vi "LED_Scaled_Output.vi"(8 "Number of LEDs":i32=8, 9 "Range Bottom":dbl, 10 "Range Top":dbl=10.0, 11 "Sensor Input":dbl) -> (1 "Out of Range":bool, 3 "Output (bool)":bool[](array[boolean]), 4 "LEDs to light":dbl, 6 "Resolution":dbl)   [LabVIEW 2013]
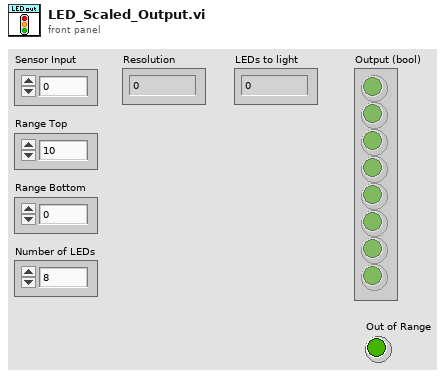
[diagram p1: front panel]
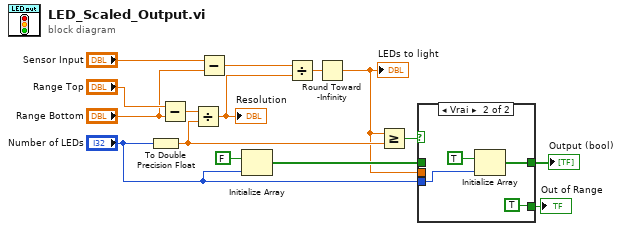
[diagram p0: block diagram]
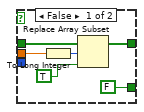
[diagram p2: hidden frame]
diagram:
  n1 = To Double Precision Float(number="Number of LEDs") -> (double precision float=w8:dbl)
  n2 = Subtract(x="Range Top", y="Range Bottom") -> (x-y=w13:dbl)
  n3 = Divide(x=w13, y=w8) -> (x/y=w12:dbl)
  "Resolution" <- w12
  n4 = Subtract(x="Sensor Input", y="Range Bottom") -> (x-y=w2:dbl)
  n5 = Initialize Array(FALSE, "Number of LEDs") -> (w10:bool[])
  n6 = Divide(x=w2, y=w12) -> (x/y=w11:dbl)
  n7 = Round Toward -Infinity(1:w11) -> (0:w5:dbl)
  "LEDs to light" <- w5
  n8 = Greater Or Equal?(x=w5, y=w8) -> (x >= y?=w9:bool)
  n9 = case shown="Vrai" w9 {
    tunnel: w10 -> [w20 _]
    tunnel: [w19 w24] -> w7
    tunnel: "Number of LEDs" -> [_ w23]
    tunnel: w5 -> [w18 _]
    tunnel: [FALSE ("new element/subarray") TRUE] -> w4
    frame False {
      n10 = To Long Integer(number=w18) -> (32bit integer=w17:i32)
      n11 = Replace Array Subset(array=w20, new element=TRUE ("new element/subarray"), index=w17) -> (w19:bool[])
    }
    frame True {
      n12 = Initialize Array(TRUE, w23) -> (w24:bool[])
    }
  }
  "Output (bool)" <- w7
  "Out of Range" <- w4
